vi "恢复参数.vi"(8 "仪器公式":T1(array[cluster]), 9 "量程参数":T2(array[cluster]), 10 "试剂容量参数":T3, 11 "外设参数":T4) -> (3 "恢复结果":string)   [LabVIEW 2016, in "斯坦道总磷.lvlib"]
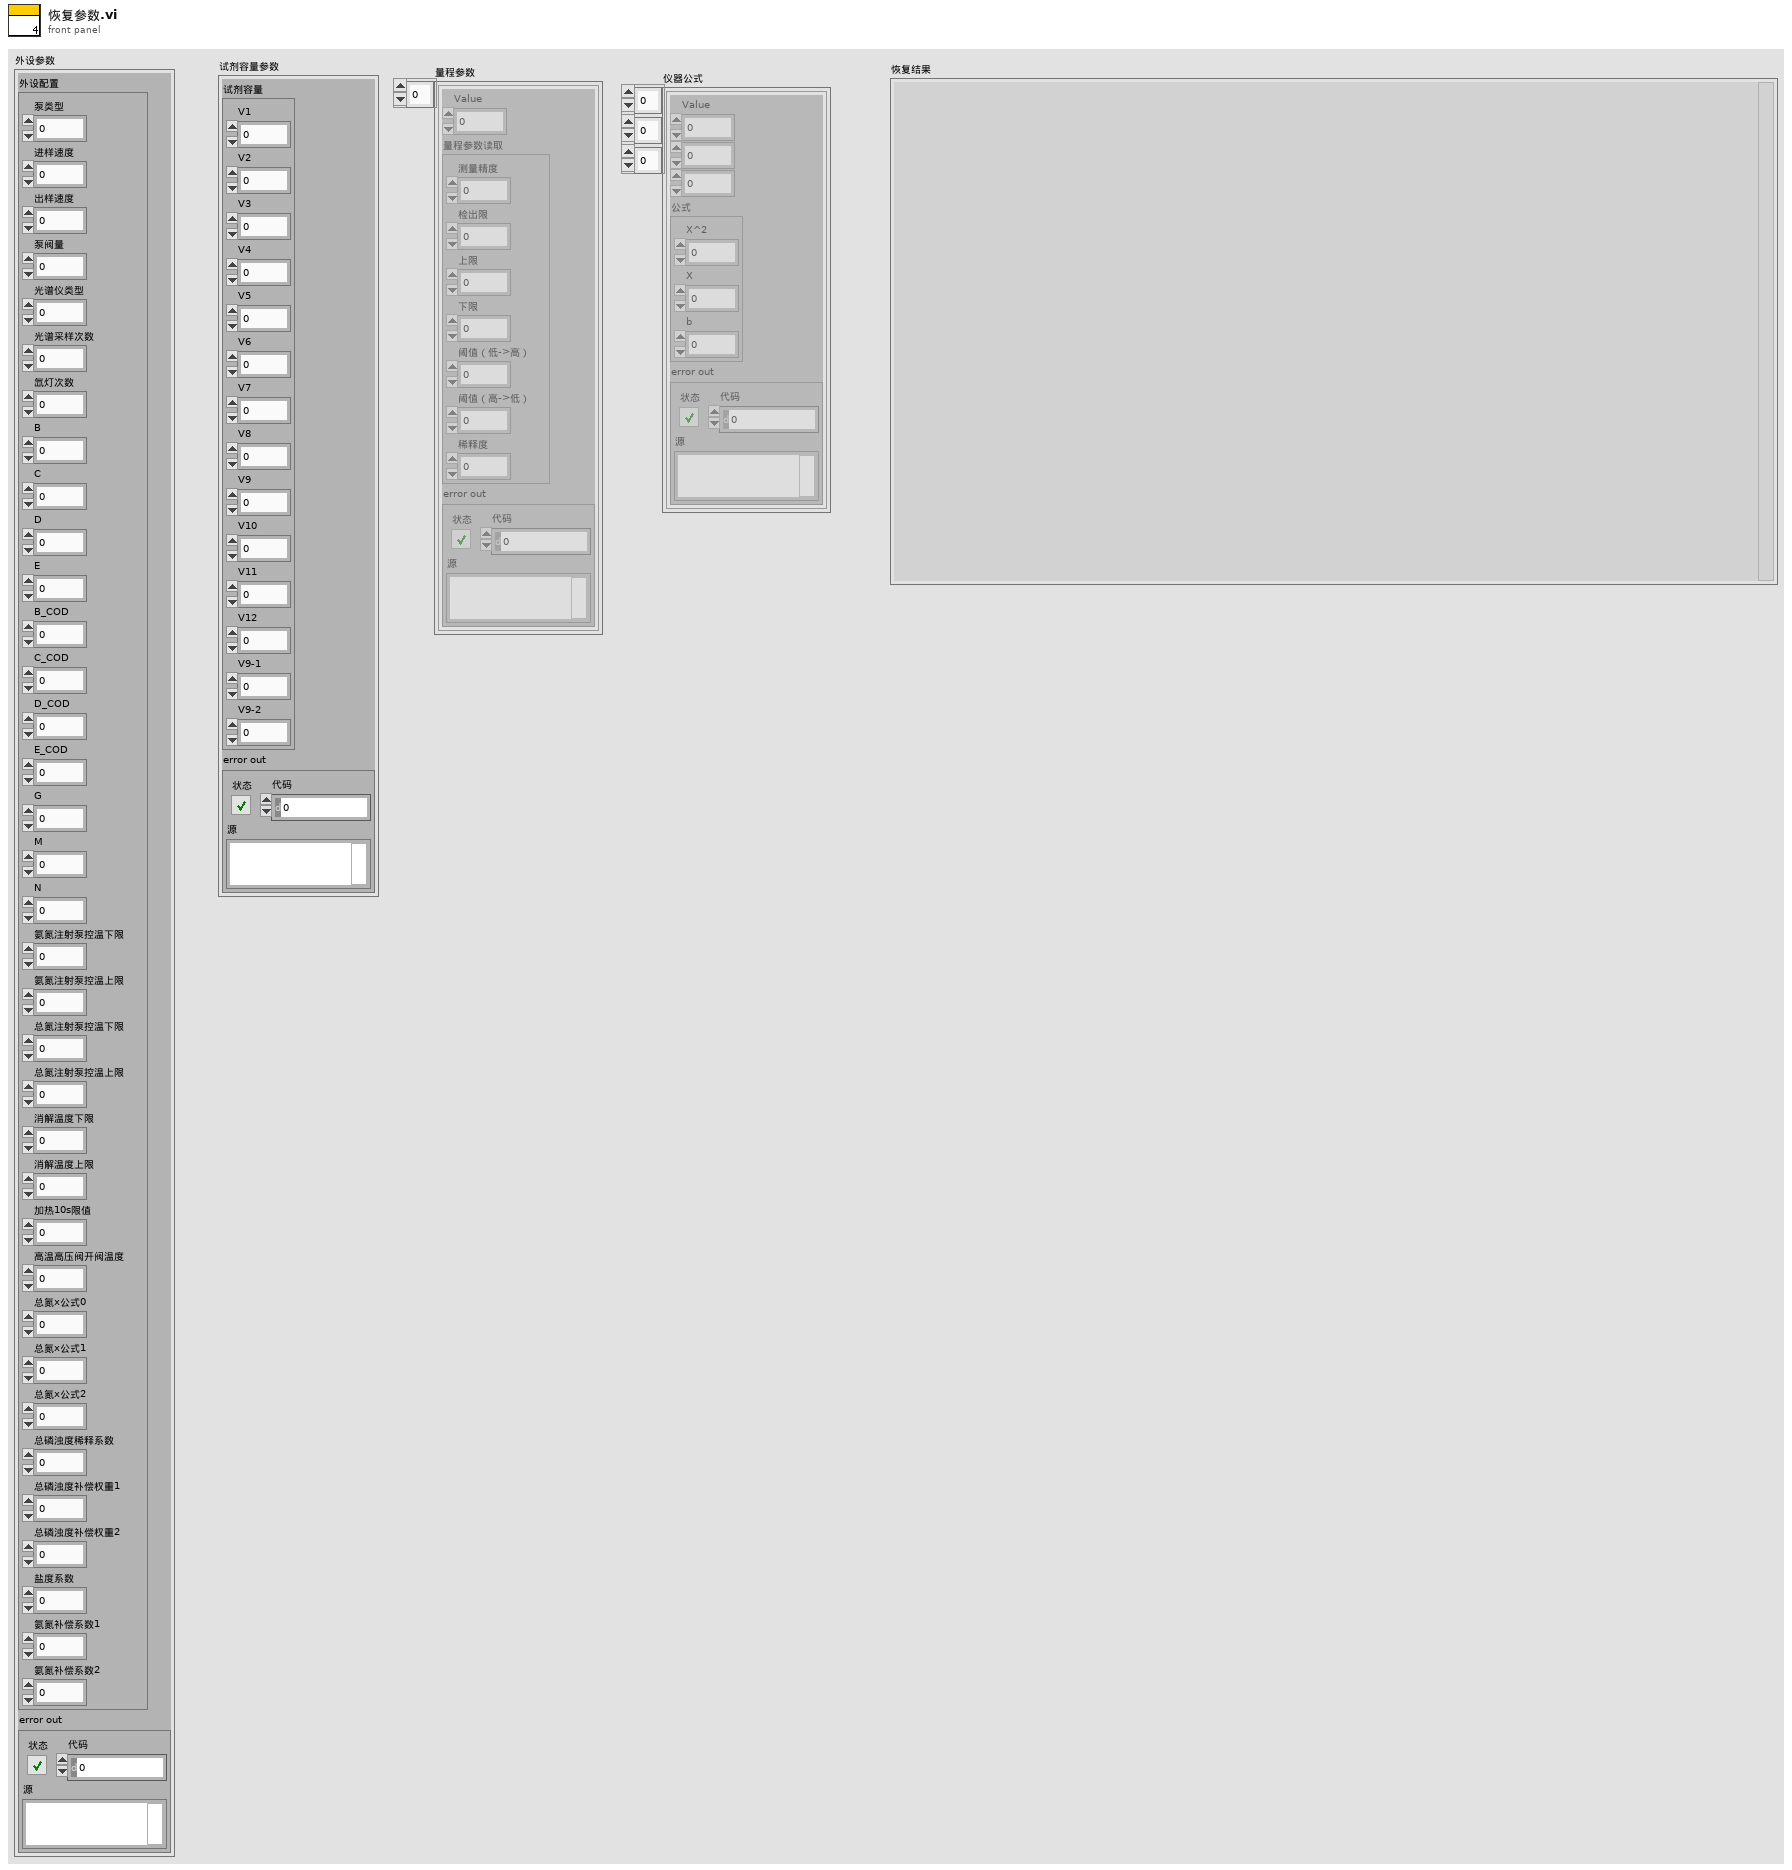
[diagram p1: front panel]
types:
  T1 = cluster{"Value":u16, i32, i32, "公式":cluster{"X^2":dbl, "X":dbl, "b":dbl}, "error out":errorcluster}[][][]
  T2 = cluster{"Value":u16, "量程参数读取":cluster{"测量精度":u16, "检出限":dbl, "上限":dbl, "下限":dbl, "阈值（低->高）":dbl, "阈值（高->低）":dbl, "稀释度":dbl}, "error out":errorcluster}[]
  T3 = cluster{"试剂容量":cluster{"V1":sgl, "V2":sgl, "V3":sgl, "V4":sgl, "V5":sgl, "V6":sgl, "V7":sgl, "V8":sgl, "V9":sgl, "V10":sgl, "V11":sgl, "V12":sgl, "V9-1":sgl, "V9-2":sgl}, "error out":errorcluster}
  T4 = cluster{"外设配置":cluster{"泵类型":u8, "进样速度":u32, "出样速度":u32, "泵阀量":u8, "光谱仪类型":u8, "光谱采样次数":u8, "氙灯次数":u8, "B":u16, "C":u16, "D":u16, "E":u16, "B_COD":u16, "C_COD":u16, "D_COD":u16, "E_COD":u16, "G":u16, "M":u16, "N":u16, "氨氮注射泵控温下限":sgl, "氨氮注射泵控温上限":sgl, "总氮注射泵控温下限":sgl, "总氮注射泵控温上限":sgl, "消解温度下限":sgl, "消解温度上限":sgl, "加热10s限值":sgl, "高温高压阀开阀温度":sgl, "总氮x公式0":u8, "总氮x公式1":sgl, "总氮x公式2":sgl, "总磷浊度稀释系数":sgl, "总磷浊度补偿权重1":sgl, "总磷浊度补偿权重2":sgl, "盐度系数":sgl, "氨氮补偿系数1":sgl, "氨氮补偿系数2":sgl}, "error out":errorcluster}
  T5 = enum16{"恢复外设参数", "恢复试剂容量参数", "恢复量程参数", "恢复仪器公式", "结束"}
  T6 = cluster{"泵类型":u8, "进样速度":u32, "出样速度":u32, "泵阀量":u8, "光谱仪类型":u8, "光谱采样次数":u8, "氙灯次数":u8, "B":u16, "C":u16, "D":u16, "E":u16, "B_COD":u16, "C_COD":u16, "D_COD":u16, "E_COD":u16, "G":u16, "M":u16, "N":u16, "氨氮注射泵控温下限":sgl, "氨氮注射泵控温上限":sgl, "总氮注射泵控温下限":sgl, "总氮注射泵控温上限":sgl, "消解温度下限":sgl, "消解温度上限":sgl, "加热10s限值":sgl, "高温高压阀开阀温度":sgl, "总氮x公式0":u8, "总氮x公式1":sgl, "总氮x公式2":sgl, "总磷浊度稀释系数":sgl, "总磷浊度补偿权重1":sgl, "总磷浊度补偿权重2":sgl, "盐度系数":sgl, "氨氮补偿系数1":sgl, "氨氮补偿系数2":sgl}
  T7 = cluster{"V1":sgl, "V2":sgl, "V3":sgl, "V4":sgl, "V5":sgl, "V6":sgl, "V7":sgl, "V8":sgl, "V9":sgl, "V10":sgl, "V11":sgl, "V12":sgl, "V9-1":sgl, "V9-2":sgl}
  T8 = cluster{"测量精度":u16, "检出限":dbl, "上限":dbl, "下限":dbl, "阈值（低->高）":dbl, "阈值（高->低）":dbl, "稀释度":dbl}
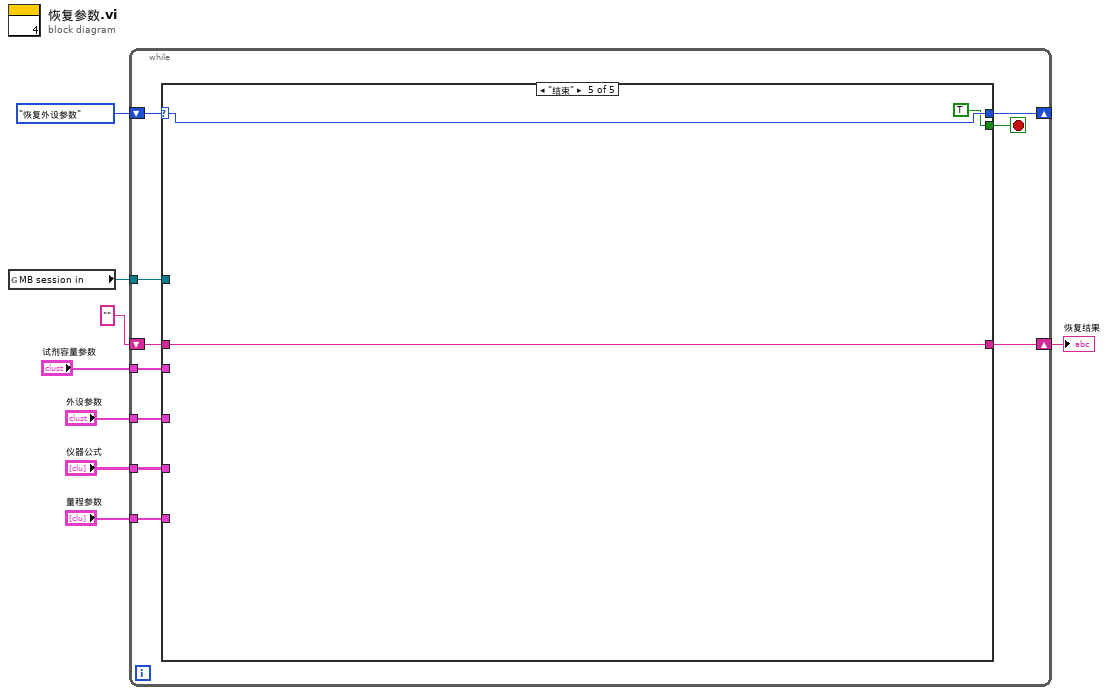
[diagram p0: block diagram]
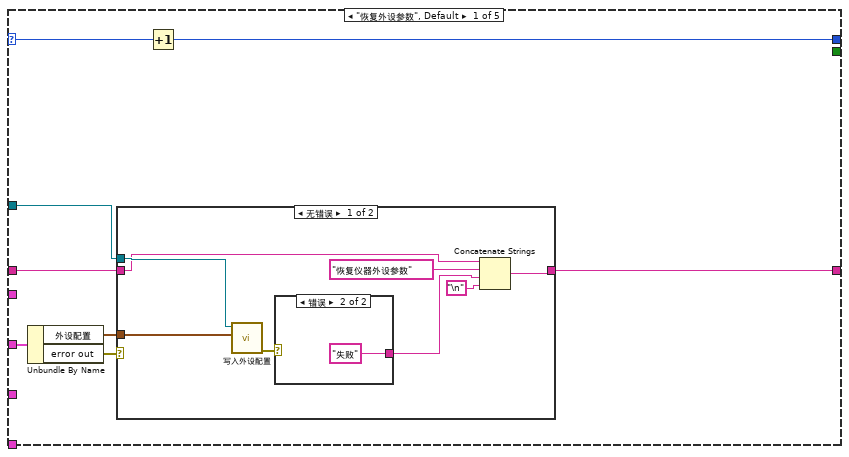
[diagram p2: hidden frame]
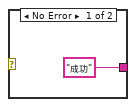
[diagram p3: hidden frame]
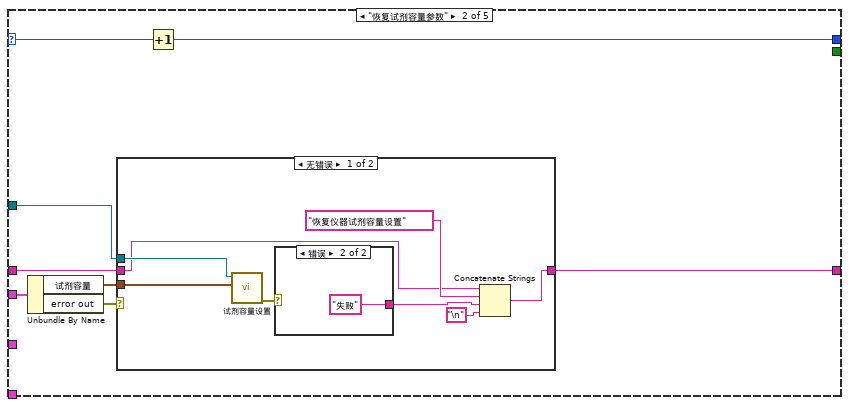
[diagram p5: hidden frame]
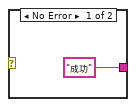
[diagram p6: hidden frame]
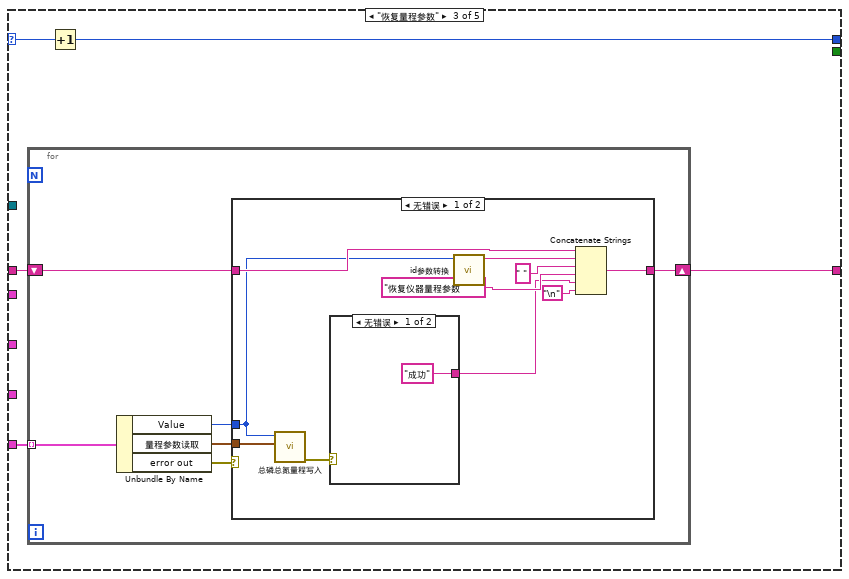
[diagram p8: hidden frame]
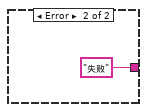
[diagram p9: hidden frame]
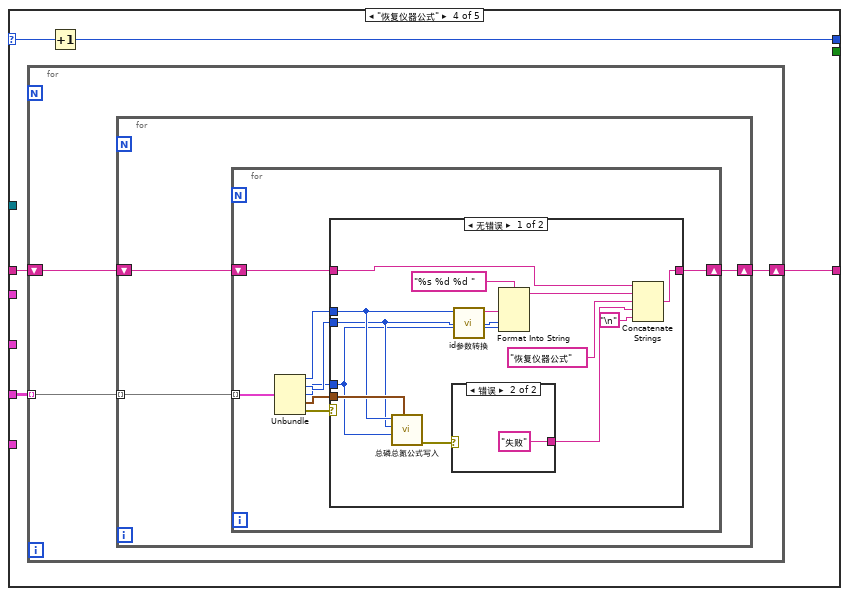
[diagram p11: hidden frame]
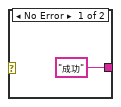
[diagram p12: hidden frame]
diagram:
  n1 = global read "VAR总磷总氮全局变量.vi" "MB session in"() -> (w5:refnum<class "MB_Master.lvclass">)
  n2 = while {
    shift-right: [w17] -> _
    shift-left: T5."恢复外设参数" ("枚举") -> [w18]
    tunnel: "外设参数" -> [w16]
    shift-right: [w10] -> w1
    shift-left: "" -> [w15]
    tunnel: w5 -> [w14]
    tunnel: "试剂容量参数" -> [w13]
    tunnel: "量程参数" -> [w12]
    tunnel: "仪器公式" -> [w11]
    stop <- w9 stop-if-true
    n3 = case shown="\"结束\"" w18 {
      selector: w18 -> [w26 w45 w61 w85 w118]
      tunnel: [w25 w44 w60 w84 w118] -> w17
      tunnel: w16 -> [w24 _ _ _ _]
      tunnel: w15 -> [w21 w39 w58 w82 w117]
      tunnel: w14 -> [w20 w41 _ _ _]
      tunnel: w13 -> [_ w43 _ _ _]
      tunnel: w12 -> [_ _ w59 _ _]
      tunnel: w11 -> [_ _ _ w83 _]
      tunnel: [w19 w38 w57 w81 w117] -> w10
      tunnel: [_ _ _ _ TRUE] -> w9
      frame "恢复外设参数", Default {
        n4 = Unbundle By Name(w24) -> ("外设配置"=w23:T6, "error out"=w22:errorcluster)
        n5 = case shown="无错误" w22 {
          tunnel: w20 -> [w34 _]
          tunnel: w23 -> [w33 _]
          tunnel: [w29 w37] -> w19
          tunnel: w21 -> [w28 w37]
          frame No Error {
            n6 = call "写入外设配置.vi"("外设配置"=w33, "MB session in"=w34) -> ("error out"=w30:errorcluster)  [unwired: 8 in, 1 out]
            n7 = case shown="错误" w30 {
              tunnel: ["成功" "失败"] -> w31
              frame No Error {
              }
              frame Error {
              }
            }
            n8 = Concatenate Strings(w28, "恢复仪器外设参数" ("字符串"), w31, "\n") -> (w29:string)
          }
          frame Error {
          }
        }
        n9 = Increment(x=w26) -> (x+1=w25:T5)
      }
      frame "恢复试剂容量参数" {
        n10 = Unbundle By Name(w43) -> ("试剂容量"=w42:T7, "error out"=w40:errorcluster)
        n11 = case shown="无错误" w40 {
          tunnel: w42 -> [w53 _]
          tunnel: w41 -> [w52 _]
          tunnel: w39 -> [w48 w56]
          tunnel: [w47 w56] -> w38
          frame No Error {
            n12 = call "试剂容量设置.vi"("试剂容量"=w53, "MB session in"=w52) -> ("error out"=w49:errorcluster)  [unwired: 8 in, 1 out]
            n13 = case shown="错误" w49 {
              tunnel: ["成功" "失败"] -> w50
              frame No Error {
              }
              frame Error {
              }
            }
            n14 = Concatenate Strings(w48, "恢复仪器试剂容量设置" ("字符串"), w50, "\n") -> (w47:string)
          }
          frame Error {
          }
        }
        n15 = Increment(x=w45) -> (x+1=w44:T5)
      }
      frame "恢复量程参数" {
        n16 = for {
          tunnel: w59 -> [w67] mode=indexing
          shift-right: [w62] -> w57
          shift-left: w58 -> [w63]
          n17 = Unbundle By Name(w67) -> ("Value"=w65:u16, "量程参数读取"=w66:T8, "error out"=w64:errorcluster)
          n18 = case shown="无错误" w64 {
            tunnel: w66 -> [w77 _]
            tunnel: w65 -> [w71 _]
            tunnel: w63 -> [w73 w80]
            tunnel: [w72 w80] -> w62
            frame No Error {
              n19 = call "总磷总氮量程写入.vi"("量程参数写入"=w77, "测量参数"=w71) -> ("error out"=w74:errorcluster)  [unwired: 8 in]
              n20 = case shown="无错误" w74 {
                tunnel: ["成功" "失败"] -> w75
                frame No Error {
                }
                frame Error {
                }
              }
              n21 = call "id参数转换.vi"("id"=w71) -> ("table输出"=w70:string)  [unwired: 9 in, 1 out]
              n22 = Concatenate Strings(w73, w70, " " ("字符串"), "恢复仪器量程参数" ("字符串"), w75, "\n") -> (w72:string)
            }
            frame Error {
            }
          }
        }
        n23 = Increment(x=w61) -> (x+1=w60:T5)
      }
      frame "恢复仪器公式" {
        n24 = for {
          tunnel: w83 -> [w88] mode=indexing
          shift-right: [w86] -> w81
          shift-left: w82 -> [w87]
          n25 = for {
            tunnel: w88 -> [w91] mode=indexing
            shift-right: [w89] -> w86
            shift-left: w87 -> [w90]
            n26 = for {
              tunnel: w91 -> [w99] mode=indexing
              shift-right: [w92] -> w89
              shift-left: w90 -> [w93]
              n27 = Unbundle(w99) -> ("Value"=w97:u16, w96:i32, w95:i32, "公式"=w94:cluster{"X^2":dbl, "X":dbl, "b":dbl}, "error out"=w98:errorcluster)
              n28 = case shown="无错误" w98 {
                tunnel: w97 -> [w105 _]
                tunnel: w96 -> [w104 _]
                tunnel: w95 -> [w103 _]
                tunnel: w94 -> [w112 _]
                tunnel: w93 -> [w102 w115]
                tunnel: [w101 w115] -> w92
                frame No Error {
                  n29 = call "总磷总氮公式写入.vi"("公式"=w112, "量程"=w103, "测量模式"=w104, "测量参数"=w105) -> ("error out"=w106:errorcluster)  [unwired: 7 in]
                  n30 = case shown="错误" w106 {
                    tunnel: ["成功" "失败"] -> w111
                    frame No Error {
                    }
                    frame Error {
                    }
                  }
                  n31 = call "id参数转换.vi"("id"=w105) -> ("table输出"=w108:string)  [unwired: 9 in, 1 out]
                  n32 = Format Into String(format string="%s %d %d " ("格式字符串"), w108, w104, w103) -> (resulting string=w107:string)  [unwired: 2 in, 1 out]
                  n33 = Concatenate Strings(w102, w107, "恢复仪器公式" ("字符串"), w111, "\n") -> (w101:string)
                }
                frame Error {
                }
              }
            }
          }
        }
        n34 = Increment(x=w85) -> (x+1=w84:T5)
      }
      frame "结束" {
      }
    }
  }
  "恢复结果" <- w1
